vi "Format 2D Array into CharX-Separated Lines.vi"(1 "2D Matrix":dbl[][](array[numeric]), 2 "delimiter (Tab)":string) -> (0 "String":string)   [LabVIEW 2016]
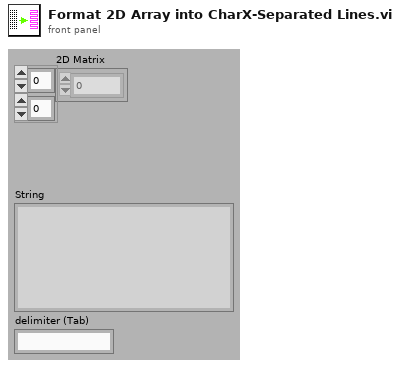
[diagram p1: front panel]
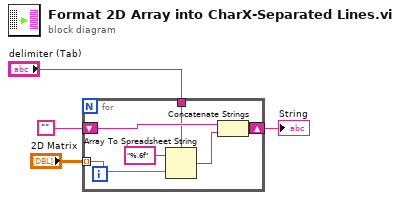
[diagram p0: block diagram]
diagram:
  n1 = for {
    tunnel: "2D Matrix" -> [w10] mode=indexing
    shift-right: [w7] -> w3
    shift-left: "" -> [w8]
    tunnel: "delimiter (Tab)" -> [w5]
    n2 = Array To Spreadsheet String(delimiter (Tab)=w5, array=w10, 3:"%.6f" ("format string")) -> (spreadsheet string=w9:string)
    n3 = Concatenate Strings(w8, w9) -> (w7:string)
  }
  "String" <- w3
